vi "BigAccDAQ.vi"() -> ()   [LabVIEW 2013]
uses:
  <vilib>/Utility/miscctls.llb/LVPointTypeDef.ctl
  <instrlib>/niScope/Controls/niScope vertical coupling.ctl
  <instrlib>/niScope/Controls/niScope trigger coupling.ctl
  <instrlib>/niScope/Controls/niScope trigger slope.ctl
  <instrlib>/niScope/Controls/niScope trigger source.ctl
  Database2.0/Public API/Dust_Event.ctl
  Database2.0/Public API/Signal.ctl
  Database2.0/Private/Controls/Role ID.ctl
  Database2.0/Private/Controls/Hardware ID.ctl
  Database2.0/Private/Controls/Estimate_source.ctl
  <instrlib>/niScope/Configure/Trigger/niScope Configure Trigger Edge.vi
  <instrlib>/niScope/Acquire/Fetch/niScope Multi Fetch Cluster.vi
  Database2.0/Private/Unused/PSU updated.vi
panel:
  out "Detectors 1 and 2":waveform(dbl)[](graph)
  in  "Write to Database?":bool
  out "PSU":waveform(dbl)(graph)
  out "Detector 3":waveform(dbl)(graph)
  out "Avg. Rate":dbl format="%#.3g"
  in  "Ref. Pos.":dbl=40.0 format="%#_13g"
  in  "Reset Count":bool
  in  "min sample rate":dbl=1000000.0 format="%.2p"
  in  "Clear Errors?":bool
  out "No. of Events":i32
  out "error out":errorcluster
  in  "stop":bool
  in  "trigger level":dbl=0.5 format="%.4f"
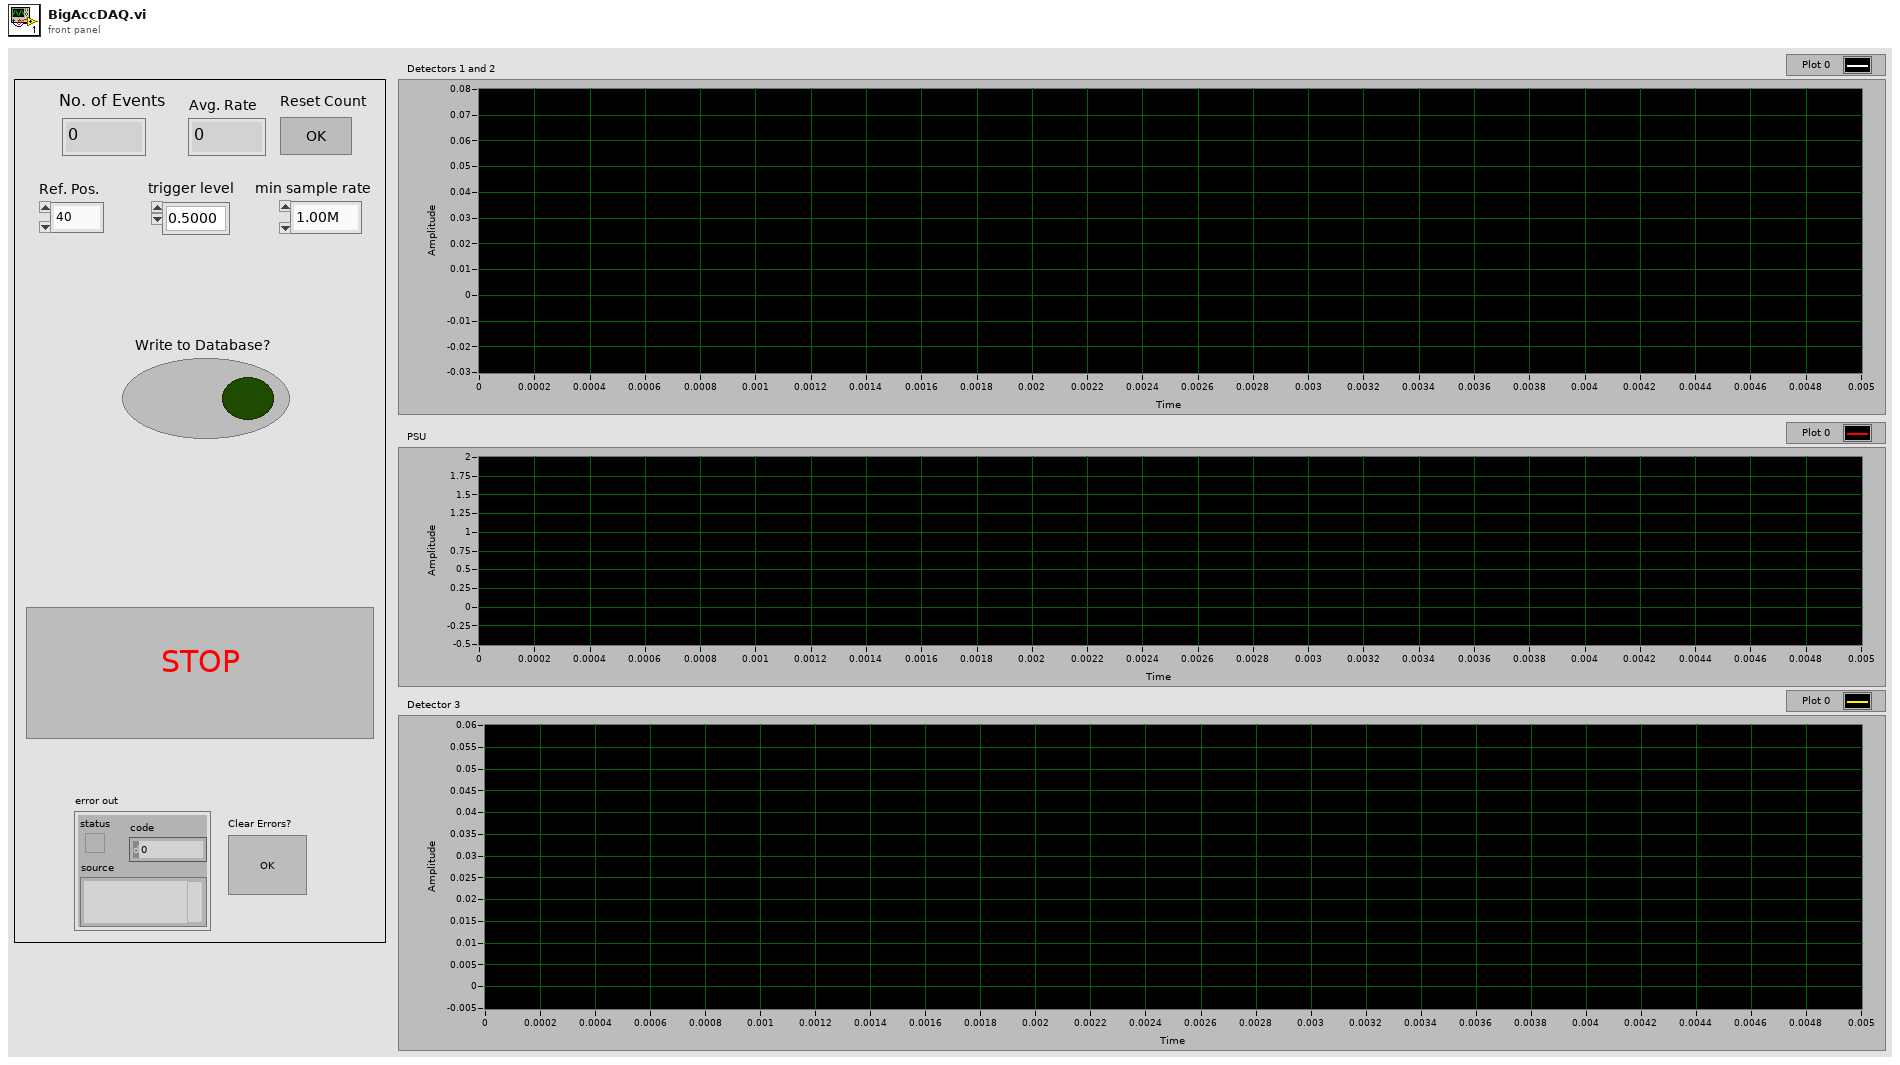
[diagram p1: front panel]
types:
  T1 = typedef "LVPointTypeDef.ctl" = cluster{"Horizontal":i16, "Vertical":i16}
  T2 = typedef "niScope trigger source.ctl" = string
  T3 = cluster{"relativeInitialX":dbl, "xIncrement":dbl, "wfm":dbl[]}[]
  T4 = typedef "Dust_Event.ctl" = cluster{"Time Stamp":timestamp, "Velocity":sgl, "Mass":sgl, "Charge":sgl, "Radius":sgl, "Array":T5[], "Dust Event ID":i64, "Passed_3rd_Detector":bool, "Estimate Source":T8, "Estimate Quality":sgl}
  T5 = typedef "Signal.ctl" = cluster{"Signal ID":i64, "Time Stamp":timestamp, "Dust Event ID":i64, "Role ID":T6, "Data":sgl[], "Signal Length":i32, "dt":sgl, "Offset":dbl, "Hardware ID":T7}
  T6 = typedef "Role ID.ctl" = enum16{"First_Detector", "Second_Detector", "Third_Detector", "LeCroy_CH1", "LeCroy_CH2", "LeCroy_CH3", "LeCroy_CH4", "PSU"}
  T7 = typedef "Hardware ID.ctl" = enum16{"Unknown", "CSA 1", "CSA 2", "CSA 3", "CSA 4", "CSA 5", "CSA 6"}
  T8 = typedef "Estimate_source.ctl" = i8
  T9 = typedef "niScope vertical coupling.ctl" = i32
  T10 = typedef "niScope trigger slope.ctl" = i32
  T11 = typedef "niScope trigger coupling.ctl" = u16
  T12 = cluster{"relativeInitialX":dbl, "xIncrement":dbl, "wfm":dbl[]}
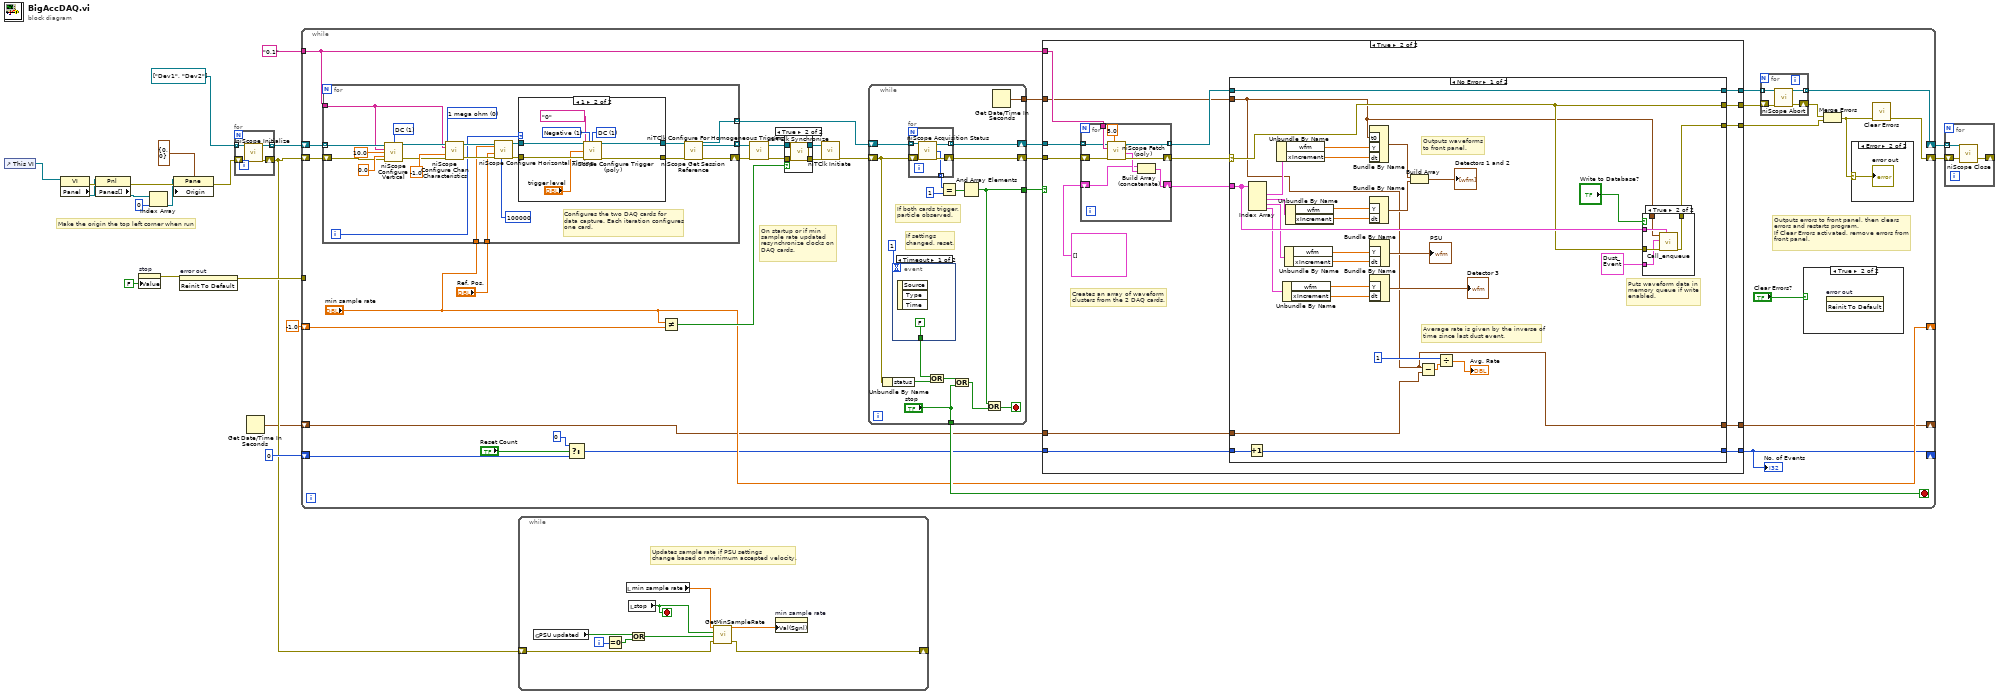
[diagram p0: block diagram]
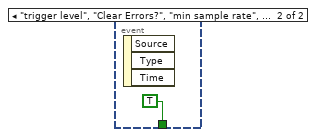
[diagram p7: hidden frame]
diagram:
  # "Make the origin the top left corner when run"
  n1 = control-ref of="This VI"() -> (w13:refnum<vi>)
  n2 = property class="VI"(reference=w13) -> (error out=w20:errorcluster, "Panel"=w14:refnum<vi>)  [unwired: 1 in, 1 out]
  n3 = property class="Pnl"(reference=w14, error in=w20) -> (error out=w19:errorcluster, "Panes[]"=w18:refnum<vi>[])  [unwired: 1 out]
  n4 = property on="stop" class="Bool (strict)"("Value"=FALSE ("stop")) -> (error out=w4:errorcluster)  [unwired: 2 in, 1 out]
  n5 = Index Array(array=w18, index=0) -> (element=w16:refnum<vi>)
  n6 = property class="Pane"(reference=w16, error in=w19, "Origin"=T1 {"Horizontal"=0, "Vertical"=0}) -> (error out=w21:errorcluster)  [unwired: 1 out]
  n7 = invoke on="error out" class="Clust (strict)" method="Reinit To Default"(error in=w4) -> (error out=w10:errorcluster)  [unwired: 2 in, 2 out]
  n8 = for {
    tunnel: [w23] -> w9 mode=indexing
    tunnel: refnum<k15>[] ["Dev1", "Dev2"] -> [w22] mode=indexing
    shift-right: [w24] -> w6
    shift-left: w21 -> [w25]
    n9 = call <instrlib>:"niScope Initialize.vi"("resource name"=w22, "error in"=w25) -> ("instrument handle"=w23:refnum<k15>, "error out"=w24:errorcluster)  [unwired: 12 in]
  }
  n10 = Get Date/Time In Seconds() -> (seconds since 1Jan1904=w3:timestamp)
  n11 = while {
    tunnel: "0,1" ("channels") -> [w37]
    shift-right: [w47] -> w2
    shift-left: w9 -> [w59]
    shift-right: [w46] -> w1
    shift-left: w6 -> [w60]
    shift-right: [w28] -> _
    shift-left: 0 -> [w31]
    tunnel: w10 -> [_]
    shift-right: ["min sample rate"] -> _
    shift-left: -1.0 ("min sample rate") -> [w42]
    shift-right: [w33] -> _
    shift-left: w3 -> [w35]
    stop <- w43 stop-if-true
    # "Outputs errors to front panel, then clears \nerrors and restarts program. \nIf Clear Errors activated, remove errors from \nfront panel."
    # "On startup or if min \nsample rate updated\nresynchronize clocks on \nDAQ cards."
    n12 = for {
      tunnel: w59 -> [w89] mode=indexing
      tunnel: [w76] -> w41 mode=indexing
      tunnel: w37 -> [w78]
      shift-right: [w74] -> w52
      shift-left: w60 -> [w90]
      tunnel: [w73] -> w53 mode=indexing
      tunnel: "min sample rate" -> [w71]
      tunnel: "Ref. Pos." -> [w72]
      i -> [w77]
      w88 = u32 0 items=["1 mega ohm"=0, "50 ohms"=2] ("input impedance")
      w91 = T9 1 items=["AC", "DC", "Ground"] ("vertical coupling")
      # "Configures the two DAQ cards for \ndata capture. Each iteration configures\none card."
      n13 = call <instrlib>:"niScope Configure Vertical.vi"("instrument handle"=w89, "vertical coupling"=w91, "channels"=w78, "vertical range"=10.0, "vertical offset"=0.0, "error in"=w90) -> ("instrument handle out"=w85:refnum<k15>, "error out"=w86:errorcluster)  [unwired: 8 in]
      n14 = call <instrlib>:"niScope Configure Chan Characteristics.vi"("instrument handle"=w85, "channels"=w78, "input impedance"=w88, "maximum input frequency"=-1.0, "error in"=w86) -> ("instrument handle out"=w82:refnum<k15>, "error out"=w83:errorcluster)  [unwired: 9 in]
      n15 = call <instrlib>:"niScope Configure Horizontal Timing.vi"("instrument handle"=w82, "min sample rate"=w71, "reference position"=w72, "error in"=w83, "min record length"=100000) -> ("instrument handle out"=w81:refnum<k15>, "error out"=w80:errorcluster)  [unwired: 9 in]
      n16 = case shown="1" w77 {
        tunnel: w81 -> [w95 w103]
        tunnel: w80 -> [w94 w102]
        tunnel: [w95 w97] -> w79
        tunnel: [w94 w96] -> w75
        frame 0, Default {
        }
        frame 1 {
          w100 = T10 1 items=["Positive", "Negative"] ("trigger slope")
          w101 = T11 1 items=["AC"=0, "DC"=1, "HF Reject"=3, "LF Reject"=4, "AC Plus HF Reject"=1001] ("trigger coupling")
          n17 = call-poly <instrlib>:"niScope Configure Trigger (poly).vi"("instrument handle"=w103, "trigger slope"=w100, "trigger coupling"=w101, "trigger source"=T2 "0", "trigger level"="trigger level", "error in"=w102) -> ("instrument handle out"=w97:refnum<k15>, "error out"=w96:errorcluster)  [unwired: 8 in]
        }
      }
      n18 = call <instrlib>:"niScope Get Session Reference.vi"("instrument handle"=w79, "error in"=w75) -> ("instrument handle out"=w76:refnum<k15>, "session reference"=w73:refnum<k20>, "error out"=w74:errorcluster)  [unwired: 11 in]
    }
    n19 = Select(t=0, s="Reset Count", f=w31) -> (s? t:f=w34:i32)
    n20 = Not Equal?(x="min sample rate", y=w42) -> (x != y?=w45:bool)
    n21 = call <instrlib>:"niTClk Configure For Homogeneous Triggers.vi"("error in (no error)"=w52, "sessions"=w53) -> ("error out"=w50:errorcluster, "sessions out"=w51:refnum<k20>[])  [unwired: 8 in]
    n22 = case shown="True" w45 {
      tunnel: w51 -> [w62 w66]
      tunnel: w50 -> [w61 w65]
      tunnel: [w62 w64] -> w49
      tunnel: [w61 w63] -> w48
      frame False {
      }
      frame True {
        n23 = call <instrlib>:"niTClk Synchronize.vi"("error in (no error)"=w65, "sessions"=w66) -> ("error out"=w63:errorcluster, "sessions out"=w64:refnum<k20>[])  [unwired: 8 in]
      }
    }
    n24 = call <instrlib>:"niTClk Initiate.vi"("error in (no error)"=w48, "sessions"=w49) -> ("error out"=w32:errorcluster)  [unwired: 8 in, 1 out]
    n25 = while {
      shift-right: [w186] -> w56
      shift-left: w41 -> [w187]
      shift-right: [w178] -> w55
      shift-left: w32 -> [w175]
      tunnel: [w174] -> w54
      tunnel: [w180] -> w36
      tunnel: ["stop"] -> w43
      stop <- w177 stop-if-true
      # "If settings \nchanged, reset."
      # "If both cards trigger,\nparticle observed."
      n26 = Unbundle By Name(w175) -> ("status"=w172:bool)
      n27 = event shown="[0] Timeout" {
        selector: _ -> [_ _]
        dyn-events: _ -> [_ _]
        timeout: 1 -> [_ _]
        tunnel: [FALSE TRUE] -> w173
        event Timeout {
          n28 = event-data() -> ()  [unwired: 1 in, 3 out]
        }
        event "trigger level", "Clear Errors?", "min sample rate", "Reset Count", "Ref. Pos.": Value Change {
          n29 = event-data() -> ()  [unwired: 1 in, 3 out]
        }
      }
      n30 = for {
        tunnel: w187 -> [w192] mode=indexing
        tunnel: [w189] -> w186 mode=indexing
        tunnel: [w188] -> w185 mode=indexing
        shift-right: [w190] -> w178
        shift-left: w175 -> [w191]
        n31 = call <instrlib>:"niScope Acquisition Status.vi"("instrument handle"=w192, "error in"=w191) -> ("instrument handle out"=w189:refnum<k15>, "acquisition status"=w188:i32, "error out"=w190:errorcluster)  [unwired: 11 in]
      }
      n32 = Or(x=w173, y=w172) -> (x .or. y?=w182:bool)
      n33 = Equal?(x=w185, y=1) -> (x = y?=w181:bool[])
      n34 = Or(x=w182, y="stop") -> (x .or. y?=w176:bool)
      n35 = And Array Elements(Boolean array=w181) -> (logical AND=w174:bool)
      n36 = Or(x=w174, y=w176) -> (x .or. y?=w177:bool)
      n37 = Get Date/Time In Seconds() -> (seconds since 1Jan1904=w180:timestamp)
    }
    n38 = case shown="True" w54 {
      tunnel: [w107 w111] -> w29
      tunnel: [w104 w109] -> w26
      tunnel: w56 -> [w107 w122]
      tunnel: w55 -> [w104 w121]
      tunnel: [w104 w110] -> w30
      tunnel: w37 -> [_ w116]
      tunnel: w36 -> [_ w115]
      tunnel: w35 -> [w105 w114]
      tunnel: w34 -> [w106 w113]
      tunnel: [w106 w112] -> w28
      tunnel: [w105 w108] -> w33
      frame False {
      }
      frame True {
        # "Creates an array of waveform \nclusters from the 2 DAQ cards."
        n39 = for {
          tunnel: w116 -> [w171]
          tunnel: [w169] -> w118 mode=indexing
          tunnel: w122 -> [w167] mode=indexing
          shift-right: [w164] -> w117
          shift-left: T3 [] ("waveform") -> [w163]
          shift-right: [w168] -> w119
          shift-left: w121 -> [w166]
          n40 = call-poly <instrlib>:"niScope Fetch (poly).vi"("timeout"=5.0, "error in"=w166, "channels"=w171, "instrument handle"=w167) -> ("error out"=w168:errorcluster, "waveform"=w165:T3, "instrument handle out"=w169:refnum<k15>)  [unwired: 4 in, 1 out]
          n41 = Build Array (concatenate)(w163, w165) -> (w164:T3)
        }
        n42 = case shown="No Error" w119 {
          selector: w119 -> [w142 w162]
          tunnel: w117 -> [w146 _]
          tunnel: w118 -> [w144 w161]
          tunnel: [w144 w161] -> w111
          tunnel: [w145 w162] -> w109
          tunnel: w113 -> [w143 w160]
          tunnel: [w137 w160] -> w112
          tunnel: [w142 w162] -> w110
          tunnel: w115 -> [w135 _]
          tunnel: w114 -> [w126 w159]
          tunnel: [w135 w159] -> w108
          frame No Error {
            # "Puts waveform data in\nmemory queue if write \nenabled."
            # "Outputs waveforms\nto front panel."
            # "Average rate is given by the inverse of \ntime since last dust event."
            n43 = Increment(x=w143) -> (x+1=w137:i32)
            n44 = Index Array(array=w146) -> (element #1=w152:T12, element #2=w151:T12, element #3=w141:T12, element #4=w140:T12)  [unwired: 4 in]
            n45 = Unbundle By Name(w152) -> ("wfm"=w134:dbl[], "xIncrement"=w133:dbl)
            n46 = Unbundle By Name(w140) -> ("wfm"=w129:dbl[], "xIncrement"=w128:dbl)
            n47 = Unbundle By Name(w141) -> ("wfm"=w130:dbl[], "xIncrement"=w127:dbl)
            n48 = Unbundle By Name(w151) -> ("wfm"=w132:dbl[], "xIncrement"=w131:dbl)
            n49 = Bundle By Name("t0"=w135, "Y"=w134, "dt"=w133) -> (w150:waveform(dbl))  [unwired: 1 in]
            n50 = Bundle By Name("Y"=w132, "dt"=w131) -> (w149:waveform(dbl))  [unwired: 1 in]
            n51 = Bundle By Name("Y"=w130, "dt"=w127) -> (→"PSU":waveform(dbl))  [unwired: 1 in]
            n52 = Bundle By Name("Y"=w129, "dt"=w128) -> (→"Detector 3":waveform(dbl))  [unwired: 1 in]
            n53 = Build Array(w150, w149) -> (→"Detectors 1 and 2":waveform(dbl)[])
            n54 = Subtract(x=w135, y=w126) -> (x-y=w124:dbl)
            n55 = Divide(x=1 ("y"), y=w124) -> (x/y=→"Avg. Rate":dbl)
            n56 = case shown="True" "Write to Database?" {
              tunnel: w146 -> [_ w158]
              tunnel: w142 -> [w153 w157]
              tunnel: [w153 w156] -> w145
              tunnel: w135 -> [_ w155]
              tunnel: T4 {"Time Stamp"=timestamp(0 s since 1904-01-01), "Velocity"=0.0, "Mass"=0.0, "Charge"=0.0, "Radius"=0.0, "Array"=[], "Dust Event ID"=0, "Passed_3rd_Detector"=FALSE, "Estimate Source"=0, "Estimate Quality"=0.0} ("Input Data") -> [_ w154]
              frame False {
              }
              frame True {
                n57 = call "Call_enqueue.vi"("Waveform"=w158, "error in"=w157, "Input Data"=w154, "seconds since 1Jan1904"=w155) -> ("error IO"=w156:errorcluster)  [unwired: 7 in]
              }
            }
          }
          frame Error {
          }
        }
      }
    }
    "No. of Events" <- w28
    n58 = for {
      shift-right: [w70] -> w27
      shift-left: w30 -> [w69]
      tunnel: [w68] -> w47 mode=indexing
      tunnel: w29 -> [w67] mode=indexing
      n59 = call <instrlib>:"niScope Abort.vi"("instrument handle"=w67, "error in"=w69) -> ("instrument handle out"=w68:refnum<k15>, "error out"=w70:errorcluster)  [unwired: 12 in]
    }
    n60 = case shown="True" "Clear Errors?" {
      frame False {
      }
      frame True {
        n61 = invoke on="error out" class="Clust (strict)" method="Reinit To Default"() -> ()  [unwired: 3 in, 3 out]
      }
    }
    n62 = Merge Errors(w27, w26) -> (w58:errorcluster)
    n63 = case shown="Error" w58 {
      selector: w58 -> [_ w195]
      frame No Error {
      }
      frame Error {
        "error out" <- w195
      }
    }
    n64 = call <vilib>:"Clear Errors.vi"("error in (no error)"=w58) -> ("error out"=w46:errorcluster)  [unwired: 6 in]
  }
  n65 = while {
    shift-right: [w196] -> _
    shift-left: w6 -> [w201]
    i -> [w204]
    stop <- w199 stop-if-true
    # "Updates sample rate if PSU settings \nchange based on minimum accepted velocity."
    n66 = global read "PSU updated.vi" "PSU updated"() -> (w203:bool)
    n67 = Equal To 0?(x=w204) -> (x = 0?=w202:bool)
    n68 = local read "min sample rate"() -> (w198:dbl)
    n69 = local read "stop"() -> (w199:bool)
    n70 = Or(x=w203, y=w202) -> (x .or. y?=w200:bool)
    n71 = call "GetMinSampleRate.vi"("error in (no error)"=w201, "True/False"=w200, "stop"=w199, "min sample rate"=w198) -> ("error out"=w196:errorcluster, "min sample rate"=w197:dbl)  [unwired: 6 in]
    n72 = property on="min sample rate" class="DigNum (strict)"("Val(Sgnl)"=w197) -> ()  [unwired: 2 in, 2 out]
  }
  n73 = for {
    tunnel: w2 -> [w207] mode=indexing
    shift-right: [w205] -> _
    shift-left: w1 -> [w206]
    n74 = call <instrlib>:"niScope Close.vi"("instrument handle"=w207, "error in"=w206) -> ("error out"=w205:errorcluster)  [unwired: 13 in]
  }
